vi "Constructor.vi"(8 "error in":errorcluster, 11 "Value":string) -> (0 "error out":errorcluster, 3 "CustomElement":refnum<class "CustomElement.lvclass">)   [LabVIEW 2021, in "ProligentXMLGenerator.lvlib" / "CustomElement.lvclass"]
uses:
  CustomElement.lvclass
  CustomElement.lvclass/CustomElement.ctl
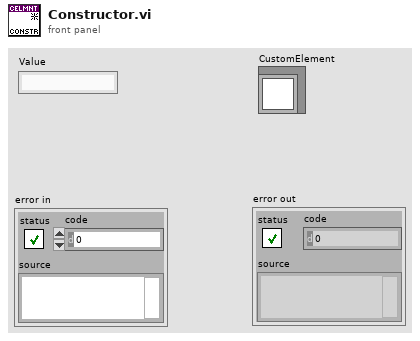
[diagram p1: front panel]
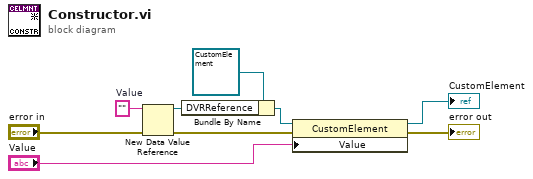
[diagram p0: block diagram]
diagram:
  w5 = ""  # Value
  n1 = New Data Value Reference(data value=w5, error in="error in") -> (data value reference=w4:refnum<data-value>, error out=w3:errorcluster)
  n2 = Bundle By Name(cluster=refnum<class "CustomElement.lvclass"> refnum ("ProligentResultProcessor:CustomElement"), "DVRReference"=w4) -> (w2:refnum<class "CustomElement.lvclass">)
  n3 = property on="Property Node" class="CustomElement"(reference=w2, error in=w3, "Value"="Value") -> (reference out=→"CustomElement":refnum<class "CustomElement.lvclass">, error out=→"error out":errorcluster)
